vi "clearSelection.vi"(8 "error in (no error)":errorcluster, 11 "CategoryListUIAdapter in":refnum<class "CategoryListUIAdapter.lvclass">) -> (0 "error out":errorcluster, 3 "CategoryListUIAdapter out":refnum<class "CategoryListUIAdapter.lvclass">)   [LabVIEW 2018, in "CategoryListUIAdapter.lvclass"]
uses:
  CategoryListUIAdapter.lvclass
  CategoryListUIAdapter.lvclass/CategoryListUIAdapter.ctl
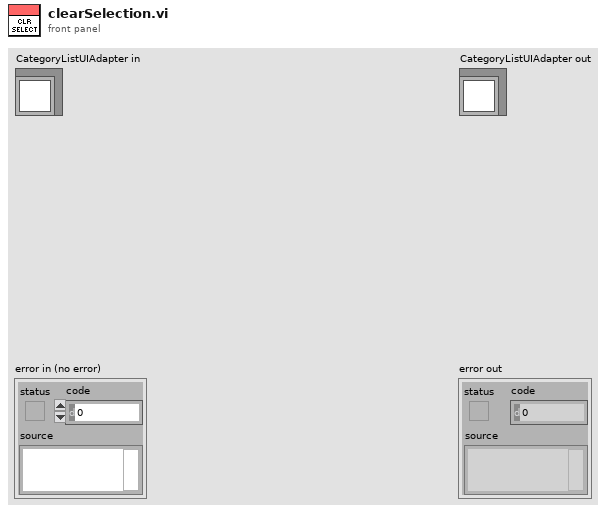
[diagram p1: front panel]
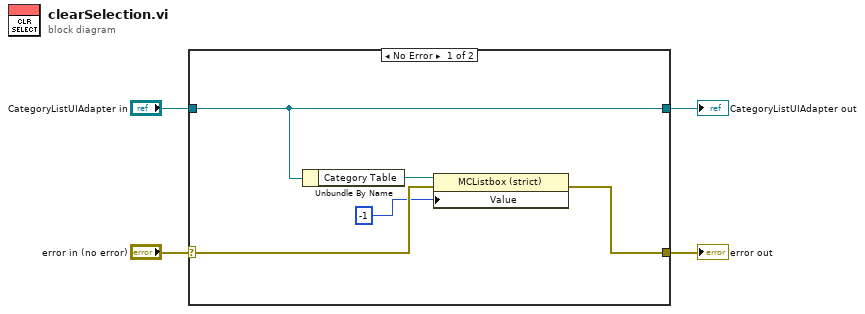
[diagram p0: block diagram]
diagram:
  n1 = case shown="No Error" "error in (no error)" {
    selector: "error in (no error)" -> [w7 w11]
    tunnel: [w6 w11] -> w3
    tunnel: [w9 w10] -> w1
    tunnel: "CategoryListUIAdapter in" -> [w9 w10]
    frame No Error {
      n2 = Unbundle By Name(w9) -> ("Category Table"=w8:refnum<vi>)
      n3 = property class="MCListbox (strict)"(reference=w8, error in=w7, "Value"=-1) -> (error out=w6:errorcluster)  [unwired: 1 out]
    }
    frame Error {
    }
  }
  "error out" <- w3
  "CategoryListUIAdapter out" <- w1
